vi "Uninit.vi"(2 "Container State":T1, 3 "Display State":T2) -> ()   [LabVIEW 2017, in "XListGraph.lvlib" / "XListGraph.xctl"]
uses:
  XListGraph.xctl
  State.ctl
  Support/def-XListGraphOper.ctl
  <vilib>/_xctls/Container State.ctl
  <vilib>/_xctls/XControlSupport.lvlib
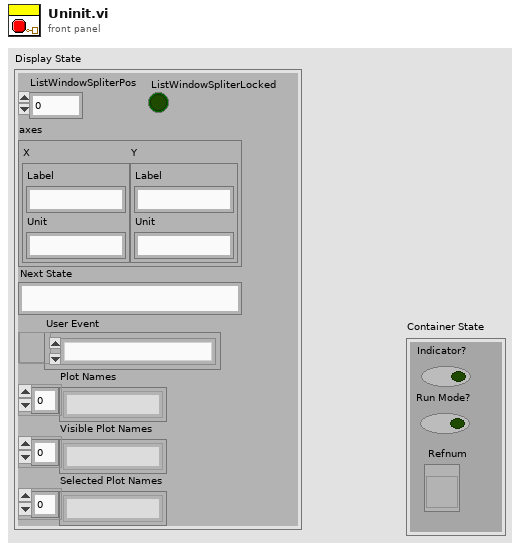
[diagram p1: front panel]
types:
  T1 = typedef "XControlSupport.lvlib/Container State.ctl" = cluster{"Indicator?":bool, "Run Mode?":bool, " Refnum":refnum<vi>}
  T2 = typedef "XListGraph.lvlib/XListGraph.xctl/State.ctl" = cluster{"ListWindowSpliterPos":i32, "ListWindowSpliterLocked":bool, "axes":cluster{"X":cluster{"Label":string, "Unit":string}, "Y":cluster{"Label":string, "Unit":string}}, "Next State":string, "User Event":refnum<user-event>, "Plot Names":string[], "Visible Plot Names":string[], "Selected Plot Names":string[]}
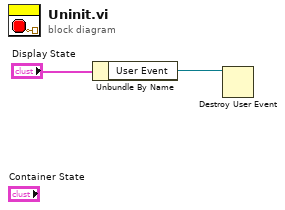
[diagram p0: block diagram]
diagram:
  n1 = Unbundle By Name("Display State") -> ("User Event"=w1:refnum<user-event>)
  n2 = Destroy User Event(user event=w1) -> ()  [unwired: 1 in, 1 out]
